vi "Close.vi"(8 "error in (no error)":errorcluster, 11 "WebDAV in":refnum<class "WebDAV.lvclass">) -> (0 "error out":errorcluster)   [LabVIEW 2016, in "RT Management.lvlib" / "WebDAV.lvclass"]
uses:
  WebDAV.lvclass
  WebDAV.lvclass/WebDAV.ctl
  Get Session.vi
  <vilib>/WebDAVClient/NI_WebDAV.lvlib
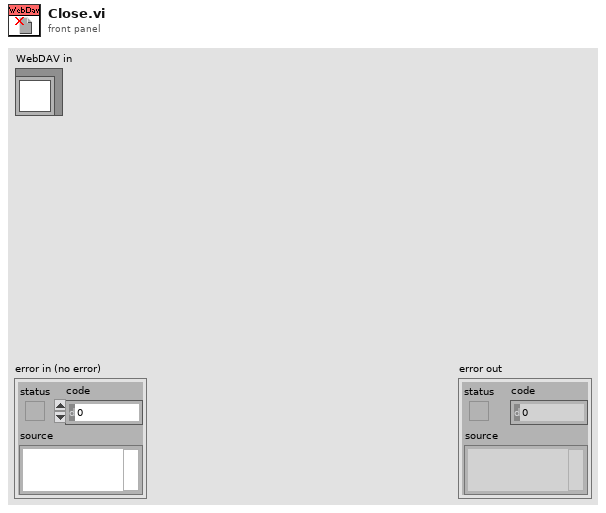
[diagram p1: front panel]
types:
  T1 = typedef "NI_WebDAV.lvlib/SessionHandle.ctl" = refnum<k1>
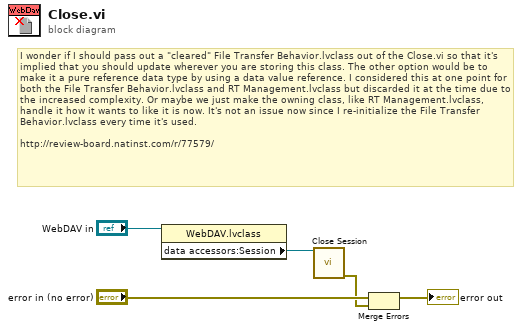
[diagram p0: block diagram]
diagram:
  # "I wonder if I should pass out a \"cleared\" File Transfer Behavior.lvclass out of the Close.vi so that it's implied that you should update wherever you are storing this class. The other option would be to make it a pure reference data type by using a data value reference. I considered this at one point for both the File Transfer Behavior.lvclass and RT Management.lvclass but discarded it at the time due to the increased complexity. Or maybe we just make the owning class, like RT Management.lvclass, handle it how it wants to like it is now. It's not an issue now since I re-initialize the File Transfer Behavior.lvclass every time it's used.\n\nhttp://review-board.natinst.com/r/77579/"
  n1 = property class="WebDAV.lvclass"(reference="WebDAV in") -> ("data accessors:Session"=w4:T1)  [unwired: 1 in, 2 out]
  n2 = call <vilib>:"Close Session.vi"("session handle"=w4) -> ("error out"=w1:errorcluster)  [unwired: 14 in]
  n3 = Merge Errors("error in (no error)", w1) -> (→"error out":errorcluster)
